vi "查找参数.vi"() -> (3 "par name":string[](array[string]))   [LabVIEW 2011]
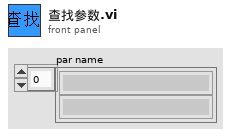
[diagram p1: front panel]
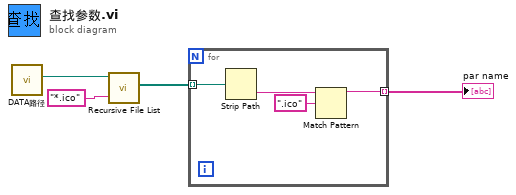
[diagram p0: block diagram]
diagram:
  n1 = call "DATA路径.vi"() -> ("DATA路径"=w4:path)  [unwired: 11 in]
  n2 = call <vilib>:"Recursive File List.vi"("pattern"="*.ico", "Folder Path"=w4) -> ("All Files in Dir"=w2:path[])  [unwired: 5 in, 4 out]
  n3 = for {
    tunnel: w2 -> [w8] mode=indexing
    tunnel: [w5] -> w1 mode=indexing
    n4 = Strip Path(path=w8) -> (name=w7:string)  [unwired: 1 out]
    n5 = Match Pattern(string=w7, regular expression=".ico" ("正则表达式")) -> (before substring=w5:string)  [unwired: 1 in, 3 out]
  }
  "par name" <- w1
